vi "LabVacHistory.vi"() -> ()   [LabVIEW 2013]
uses:
  <vilib>/Platform/TimedLoop/XDataNode/timing_clust.ctl
  <vilib>/Platform/TimedLoop/XDataNode/nitl_modes.ctl
  <vilib>/Platform/TimedLoop/XDataNode/wakeup.ctl
  <vilib>/lvdsc/historical/Read Trace (Numeric).vi
  <vilib>/platform/TimedLoop/XDataNode/XDataNode.xnode
  <vilib>/lvdsc/NI_DSC.lvlib
  <vilib>/Platform/TimedLoop/XDataNode/XDNodeRunTimeDep.lvlib
panel:
  in  "database URL":path
  out "PLOT0 PV 2":refnum<k21>
  in  "PLOT2 IDX":i32 min=0 max=8
  out "trace list":refnum<k21>[](array[refnum])
  in  "Y Scale.Mapping Mode":u8
  in  "auto update":bool
  out "PLOT1 PV":refnum<k21>
  in  "PLOT1 IDX":i32 min=-1 max=8
  out "element 3":dbl
  out "element 2":timestamp
  in  "index 2":u32
  in  "stop":bool
  out "PLOT0 PV":refnum<k21>
  in  "PLOT0 IDX":i32 min=0 max=8
  out "XY Graph":T1(graph)
  in  "time interval":T2 {"stop timestamp (now)" format="%<%X\n%x>T"; "start timestamp" format="%<%X\n%x>T"}
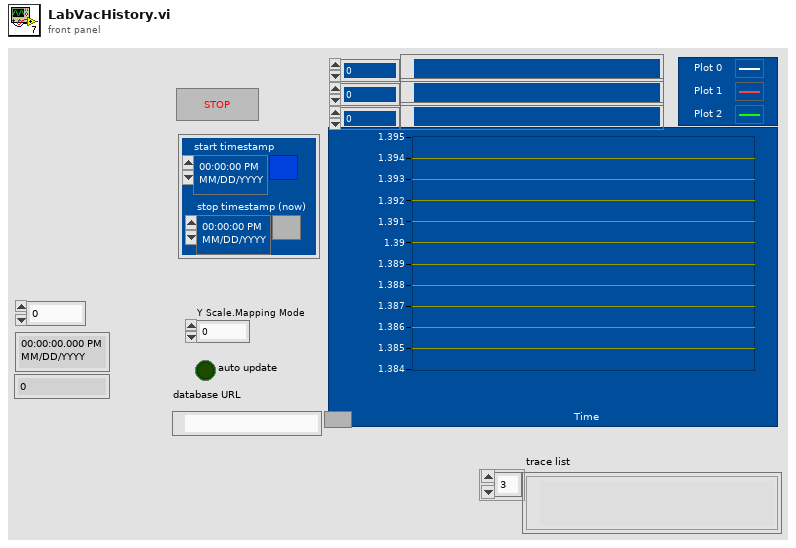
[diagram p1: front panel]
types:
  T1 = cluster{"timestamps":timestamp[], "data":dbl[]}[]
  T2 = cluster{"start timestamp":timestamp, "stop timestamp (now)":timestamp}
  T3 = typedef "XDNodeRunTimeDep.lvlib/timing_clust.ctl" = cluster{"Expected End [f-1]":u64, "Actual End [f-1]":u64, "Finished Late? [f-1]":bool, "Expected End [i-1]":u64, "Actual End [i-1]":u64, "Finished Late? [i-1]":bool, "Expected Start [i]":u64, "Actual Start [i]":u64, "Expected Start [f]":u64, "Actual Start [f]":u64, "Source Name":string, "Structure Name":string, "Period":i64, "Deadline":i64, "Offset":i64, "Start":i64, "Priority":i32, "Timeout":i32, "Mode":T4, "Wakeup Reason":T5, "Error":errorcluster, "Source Type":string, "Secondary Source Type":string, "Global End Time":u64, "Global Start Time":u64, "Frame Duration":u64, "Iteration Duration":u64, "Assigned CPU":i32, "I/O Scan Engine Mode":u32}
  T4 = typedef "XDNodeRunTimeDep.lvlib/nitl_modes.ctl" = enum32{"No Change", "Process missed periods, maintain original phase", "Discard missed periods, maintain original phase", "Process missed periods, ignore original phase", "Discard missed periods, ignore original phase"}
  T5 = typedef "XDNodeRunTimeDep.lvlib/wakeup.ctl" = enum32{"Normal", "Aborted", "Asynchronous wakeup", "Timing source error", "Timed loop error", "Timeout"}
  T6 = cluster{timestamp, "seconds since 1Jan1904":timestamp}
  T7 = cluster{"start timestamp":timestamp, "seconds since 1Jan1904":timestamp}
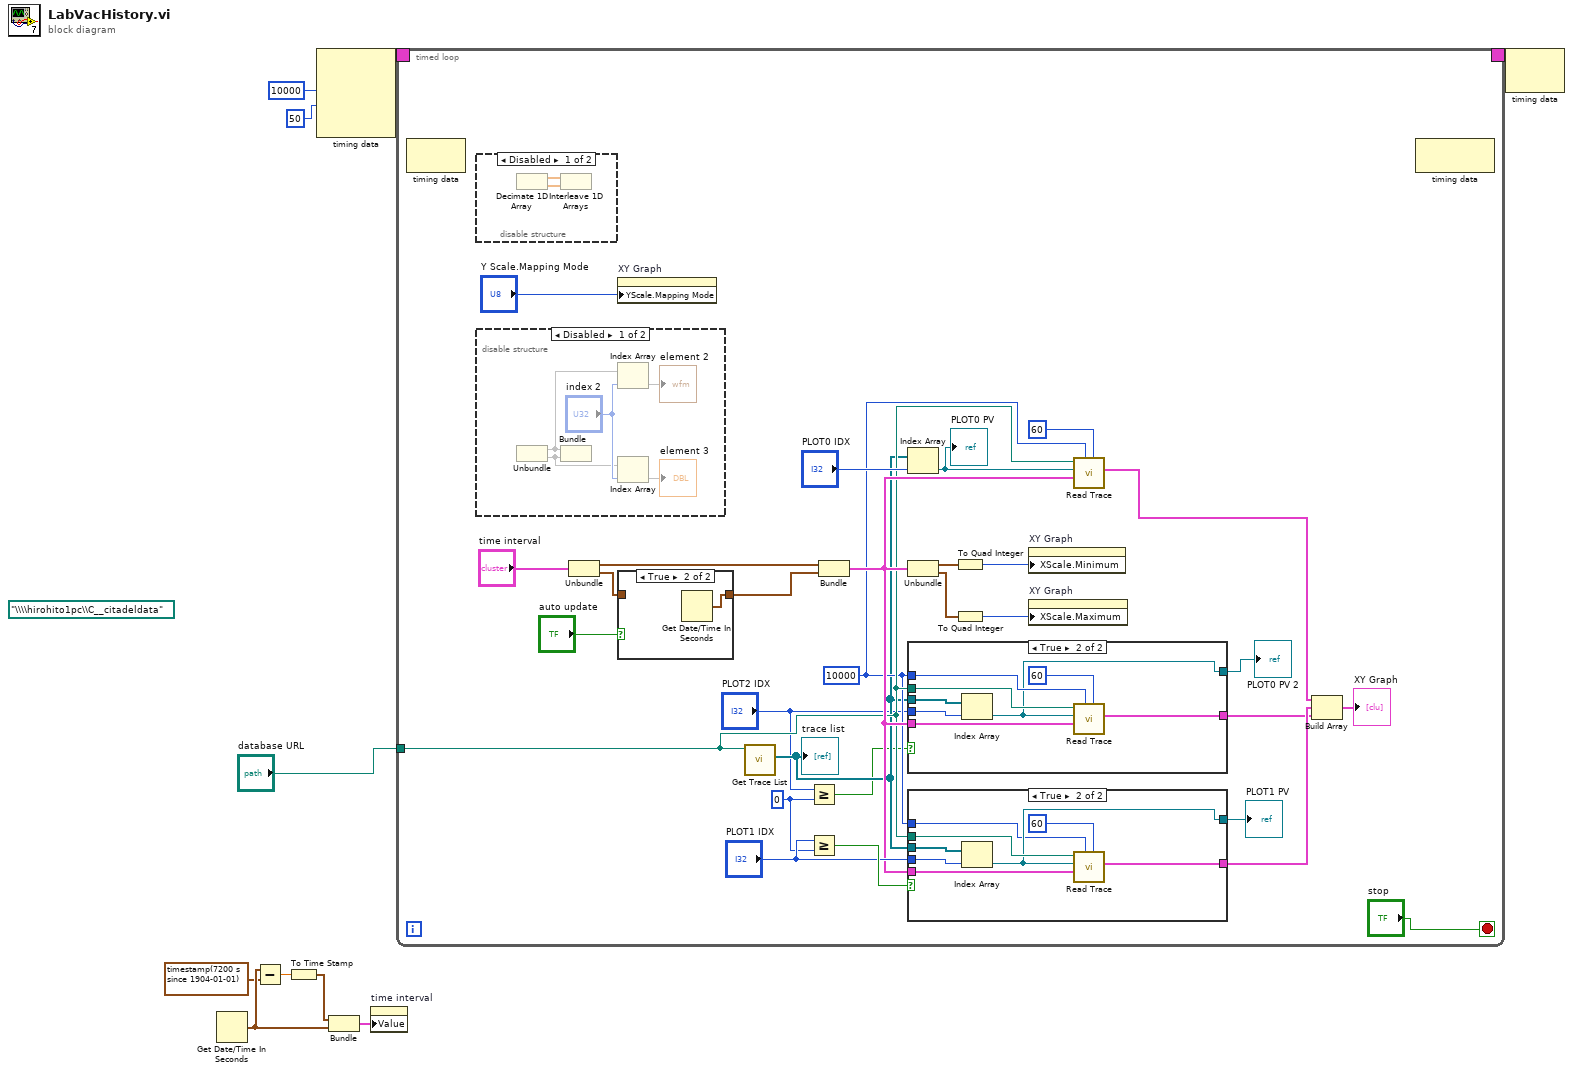
[diagram p0: block diagram]
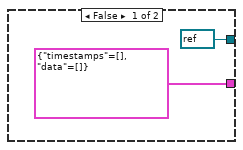
[diagram p2: hidden frame]
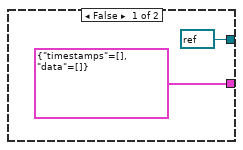
[diagram p6: hidden frame]
diagram:
  (unwired) path "\\\\hirohito1pc\\C__citadeldata" ("database URL")
  n1 = Get Date/Time In Seconds() -> (seconds since 1Jan1904=w5:timestamp)
  n2 = Subtract(x=w5, y=timestamp(7200 s since 1904-01-01)) -> (x-y=w4:dbl)
  n3 = To Time Stamp(1:w4) -> (0:w3:timestamp)
  n4 = node-c288(i64 10000 ("Period"), 50 ("Priority")) -> (w10:T3)  [unwired: 2 in]
  n5 = Bundle(w3, "seconds since 1Jan1904"=w5) -> (w6:T6)  [unwired: 1 in]
  n6 = property on="time interval" class="Clust (strict)"("Value"=w6) -> ()  [unwired: 2 in, 2 out]
  n7 = timed-loop {
    timing: w10 -> [_]
    timing-out: [_] -> w9
    tunnel: "database URL" -> [w18]
    stop <- "stop" stop-if-true
    w12 = 0 ("y")
    w17 = 10000 ("max points per trace (all)")
    n8 = node-c288() -> ()  [unwired: 1 in, 1 out]
    n9 = disable-structure shown="Disabled" {
      frame Disabled {
        n10 = Decimate 1D Array() -> (w57:dbl[], w56:dbl[])  [unwired: 1 in]
        n11 = Interleave 1D Arrays(w57, w56) -> ()  [unwired: 1 out]
      }
      frame Enabled {
      }
    }
    n12 = disable-structure shown="Disabled" {
      frame Disabled {
        n13 = Unbundle() -> (w50:cluster{"timestamps":timestamp[], "data":dbl[]}, "timestamps"=w55, "data"=w51)
        n14 = Bundle(w55, w51) -> ()  [unwired: 1 in, 1 out]
        n15 = Index Array(array=w55, index="index 2") -> (element=→"element 2")
        n16 = Index Array(array=w51, index="index 2") -> (element=→"element 3")
      }
      frame Enabled {
      }
    }
    n17 = Unbundle("time interval") -> ("start timestamp"=w31:timestamp, "stop timestamp (now)"=w23:timestamp)
    n18 = property on="XY Graph" class="XYGraph (strict)"("YScale.Mapping Mode"="Y Scale.Mapping Mode") -> ()  [unwired: 2 in, 2 out]
    n19 = case shown="True" "auto update" {
      tunnel: [w58 w59] -> w30
      tunnel: w23 -> [w58 _]
      frame False {
      }
      frame True {
        n20 = Get Date/Time In Seconds() -> (seconds since 1Jan1904=w59:timestamp)
      }
    }
    n21 = call <vilib>:"Get Trace List.vi"("database URL"=w18) -> ("trace list"=w15:refnum<k21>[])  [unwired: 6 in, 4 out]
    "trace list" <- w15
    n22 = Greater Or Equal?(x="PLOT2 IDX", y=w12) -> (x >= y?=w11:bool)
    n23 = Greater Or Equal?(x="PLOT1 IDX", y=w12) -> (x >= y?=w28:bool)
    n24 = Bundle("start timestamp"=w31, "seconds since 1Jan1904"=w30) -> (w19:T7)  [unwired: 1 in]
    n25 = Index Array(array=w15, index="PLOT0 IDX") -> (element=w38:refnum<k21>)
    "PLOT0 PV" <- w38
    n26 = Unbundle(w19) -> ("start timestamp"=w37:timestamp, "seconds since 1Jan1904"=w35:timestamp)
    n27 = case shown="True" w11 {
      tunnel: w19 -> [_ w48]
      tunnel: w18 -> [_ w47]
      tunnel: w17 -> [_ w46]
      tunnel: [refnum<k21> refnum ("Tag Name") w45] -> w16
      tunnel: w15 -> [_ w44]
      tunnel: [cluster{"timestamps":timestamp[], "data":dbl[]} {"timestamps"=[], "data"=[]} ("element") w43] -> w14
      tunnel: "PLOT2 IDX" -> [_ w42]
      frame False {
      }
      frame True {
        n28 = Index Array(array=w44, index=w42) -> (element=w45:refnum<k21>)
        n29 = call-poly <vilib>:"Read Trace.vi"("timeout (30 s)"=60, "max points per trace (all)"=w46, "time interval"=w48, "trace name"=w45, "database URL"=w47) -> ("historical trace"=w43:cluster{"timestamps":timestamp[], "data":dbl[]})  [unwired: 3 in, 3 out]
      }
    }
    "PLOT0 PV 2" <- w16
    n30 = case shown="True" w28 {
      tunnel: [cluster{"timestamps":timestamp[], "data":dbl[]} {"timestamps"=[], "data"=[]} ("element") w66] -> w27
      tunnel: w19 -> [_ w69]
      tunnel: w15 -> [_ w68]
      tunnel: "PLOT1 IDX" -> [_ w67]
      tunnel: w18 -> [_ w65]
      tunnel: [refnum<k21> refnum ("Tag Name") w64] -> w25
      tunnel: w17 -> [_ w63]
      frame False {
      }
      frame True {
        n31 = Index Array(array=w68, index=w67) -> (element=w64:refnum<k21>)
        n32 = call-poly <vilib>:"Read Trace.vi"("timeout (30 s)"=60, "max points per trace (all)"=w63, "time interval"=w69, "trace name"=w64, "database URL"=w65) -> ("historical trace"=w66:cluster{"timestamps":timestamp[], "data":dbl[]})  [unwired: 3 in, 3 out]
      }
    }
    "PLOT1 PV" <- w25
    n33 = To Quad Integer(1:w37) -> (0:w36:i64)
    n34 = To Quad Integer(1:w35) -> (0:w34:i64)
    n35 = property on="XY Graph" class="XYGraph (strict)"("XScale.Minimum"=w36) -> ()  [unwired: 2 in, 2 out]
    n36 = property on="XY Graph" class="XYGraph (strict)"("XScale.Maximum"=w34) -> ()  [unwired: 2 in, 2 out]
    n37 = call-poly <vilib>:"Read Trace.vi"("timeout (30 s)"=60, "max points per trace (all)"=w17, "time interval"=w19, "trace name"=w38, "database URL"=w18) -> ("historical trace"=w20:cluster{"timestamps":timestamp[], "data":dbl[]})  [unwired: 3 in, 3 out]
    n38 = Build Array(w20, w27, w14) -> (→"XY Graph":T1)
    n39 = node-c288() -> ()  [unwired: 1 in, 1 out]
  }
  n40 = node-c288(w9) -> ()  [unwired: 1 out]
